vi "ButtonDelay.vi"(9 "Delay(cs)":dbl, 10 "Button In":bool) -> (2 "Boolean":bool)   [LabVIEW 2013]
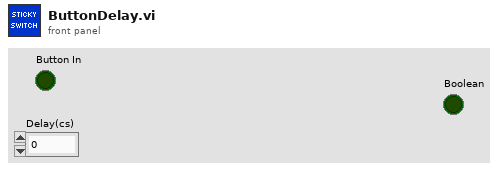
[diagram p1: front panel]
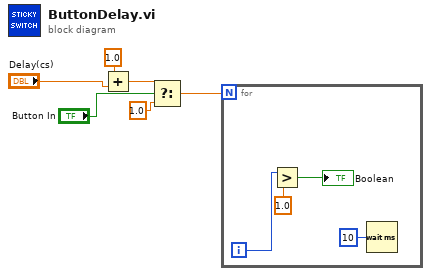
[diagram p0: block diagram]
diagram:
  n1 = Add(x=1.0, y="Delay(cs)") -> (x+y=w3:dbl)
  n2 = Select(t=w3, s="Button In", f=1.0) -> (s? t:f=w6:dbl)
  n3 = for {
    N: w6 -> [_]
    i -> [w9]
    n4 = Greater?(x=w9, y=1.0) -> (0:→"Boolean":bool)
    n5 = Wait (ms)(milliseconds to wait=u32 10) -> ()  [unwired: 1 out]
  }
